vi "add tag by line.vi"(6 "ItemNames":string[](array[string]), 7 "Properties:instance identifier":string, 8 "error in":errorcluster, 10 "TDMS datalogger configuration in":refnum<class "TDMS datalogger configuration.lvclass">, 11 "engine configuration in":refnum<class "engine configuration.lvclass">) -> (0 "error out":errorcluster, 2 "TDMS datalogger configuration out":refnum<class "TDMS datalogger configuration.lvclass">, 3 "engine configuration out":refnum<class "engine configuration.lvclass">)   [LabVIEW 2013, in "TDMS datalogger editor node.lvclass"]
uses:
  TDMS datalogger editor node.lvclass
  <vilib>/NI/Module Execution Interface/Engine Configuration/engine configuration.lvclass
  <vilib>/NI/TBM Modules/TDMS Datalogger/module/configuration/TDMS datalogger configuration.lvclass
  <vilib>/NI/Tag Bus/tag/Data Type.ctl
  <vilib>/NI/Tag Bus Module Framework/channel/channel classification.ctl
  <vilib>/NI/Tag Bus/tag/tag descriptor.lvclass
  <vilib>/NI/Tag Bus Module Framework/channel/TBM channel.lvclass
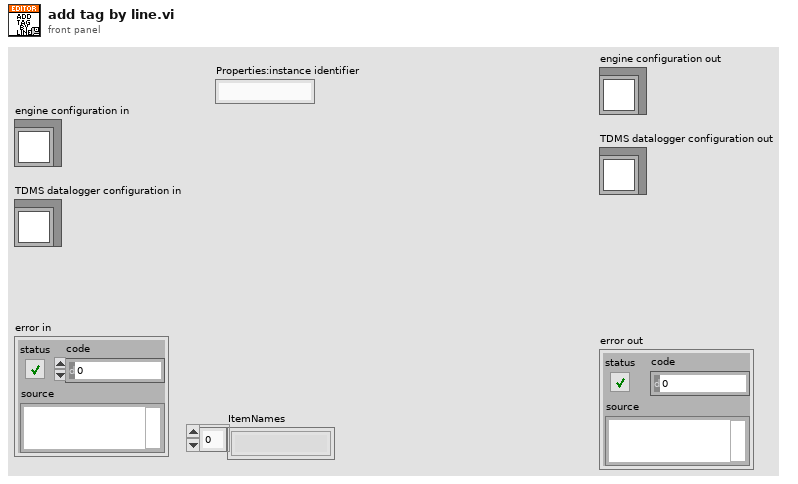
[diagram p1: front panel]
types:
  T1 = typedef "tag bus.lvlib/tag descriptor.lvclass/Data Type.ctl" = enum16{"Double", "Single", "I64", "I32", "I16", "I8", "U64", "U32", "U16", "U8", "Boolean", "String", "Array of Double", "Array of Single", "Array of I64", "Array of I32", "Array of I16", "Array of I8", "Array of U64", "Array of U32", "Array of U16", "Array of U8", "Array of Boolean", "Array of String"}
  T2 = typedef "TBM channel.lvclass/channel classification.ctl" = enum16{"input data", "output data", "processing parameter", "processing result"}
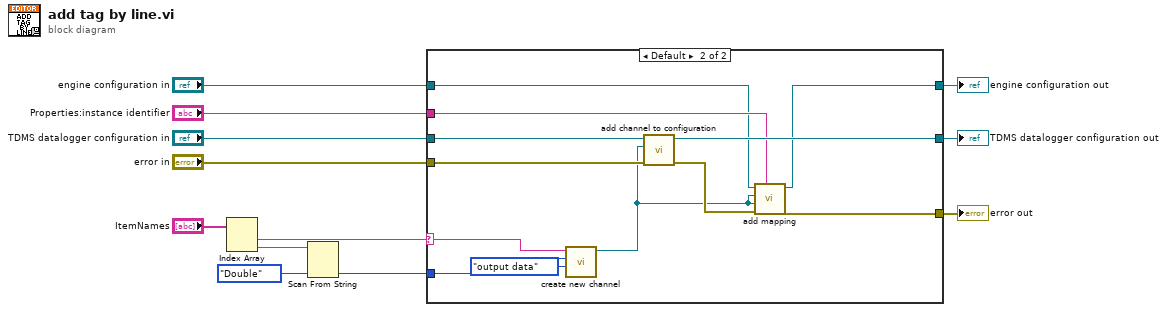
[diagram p0: block diagram]
diagram:
  n1 = Index Array(array="ItemNames") -> (element #1=w9:string, element #2=w2:string)  [unwired: 2 in]
  n2 = Scan From String(input string=w2, default 1=Data_Type."Double" ("data type")) -> (output 1=w8:T1)  [unwired: 3 in, 3 out]
  n3 = case shown="Default" w9 {
    selector: w9 -> [_ w27]
    tunnel: [w14 w22] -> w5
    tunnel: "TDMS datalogger configuration in" -> [w15 w24]
    tunnel: "error in" -> [w14 w23]
    tunnel: w8 -> [_ w26]
    tunnel: [w15 w21] -> w4
    tunnel: "engine configuration in" -> [w13 w17]
    tunnel: [w13 w18] -> w11
    tunnel: "Properties:instance identifier" -> [_ w19]
    frame "" {
    }
    frame Default {
      n4 = call <vilib>:"create new channel.vi"("channel classification"=channel_classification."output data", "data type"=w26, "channel name"=w27) -> ("channel"=w16:refnum<class "TBM channel.lvclass">)  [unwired: 8 in]
      n5 = call <vilib>:"add channel to configuration.vi"("error in"=w23, "TBM channel in"=w16, "TDMS datalogger configuration in"=w24) -> ("error out"=w20:errorcluster, "TDMS datalogger configuration out"=w21:refnum<class "TDMS datalogger configuration.lvclass">)  [unwired: 7 in]
      n6 = call <vilib>:"add mapping.vi"("owner ID"=w19, "error in"=w20, "channel"=w16, "tag descriptor"=w16, "engine configuration"=w17) -> ("error out"=w22:errorcluster, "engine configuration out"=w18:refnum<class "engine configuration.lvclass">)  [unwired: 5 in]
    }
  }
  "engine configuration out" <- w11
  "error out" <- w5
  "TDMS datalogger configuration out" <- w4
